vi "_getWorkerPath.vi"() -> (2 "Worker Path":path)   [LabVIEW 2013, in "LVAutomationListener.lvlib" / "LVAutomationListener.lvclass"]
uses:
  LVAutomationListener.lvclass
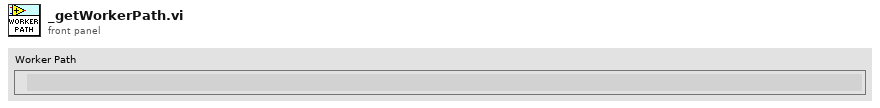
[diagram p1: front panel]
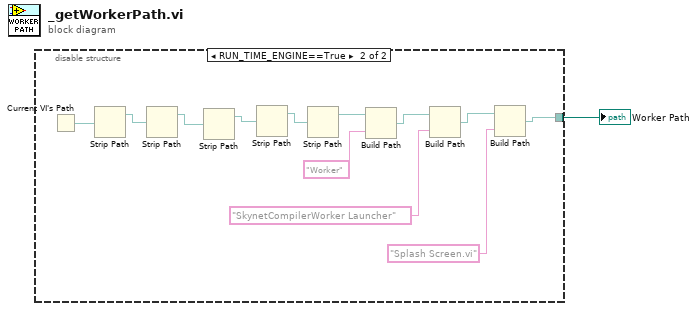
[diagram p0: block diagram]
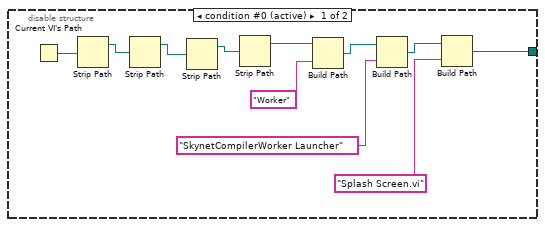
[diagram p2: hidden frame]
diagram:
  n1 = disable-structure shown="RUN_TIME_ENGINE==True" {
    disable-tunnel: [w2 w13] -> w1
    frame condition #0 (active) {
      n2 = Current VI's Path() -> (path=w12:path)
      n3 = Strip Path(path=w12) -> (stripped path=w11:path)  [unwired: 1 out]
      n4 = Strip Path(path=w11) -> (stripped path=w10:path)  [unwired: 1 out]
      n5 = Strip Path(path=w10) -> (stripped path=w9:path)  [unwired: 1 out]
      n6 = Strip Path(path=w9) -> (stripped path=w8:path)  [unwired: 1 out]
      n7 = Build Path(base path=w8, name or relative path="Worker") -> (appended path=w6:path)
      n8 = Build Path(base path=w6, name or relative path="SkynetCompilerWorker Launcher") -> (appended path=w4:path)
      n9 = Build Path(base path=w4, name or relative path="Splash Screen.vi") -> (appended path=w2:path)
    }
    frame condition #1 {
      n10 = Current VI's Path() -> (path=w22:path)
      n11 = Strip Path(path=w22) -> (stripped path=w21:path)  [unwired: 1 out]
      n12 = Strip Path(path=w21) -> (stripped path=w20:path)  [unwired: 1 out]
      n13 = Strip Path(path=w20) -> (stripped path=w19:path)  [unwired: 1 out]
      n14 = Strip Path(path=w19) -> (stripped path=w23:path)  [unwired: 1 out]
      n15 = Strip Path(path=w23) -> (stripped path=w24:path)  [unwired: 1 out]
      n16 = Build Path(base path=w24, name or relative path="Worker") -> (appended path=w17:path)
      n17 = Build Path(base path=w17, name or relative path="SkynetCompilerWorker Launcher") -> (appended path=w15:path)
      n18 = Build Path(base path=w15, name or relative path="Splash Screen.vi") -> (appended path=w13:path)
    }
  }
  "Worker Path" <- w1
